vi "Patch data preview core.vi"(6 "Global cycle number among all trials":i32, 9 "Channel to load":enum16{"Red", "Green"}(ring)) -> (1 "Image ref (montage)":T1, 3 "Next state":T2=enum."Idle")   [LabVIEW 2017]
uses:
  Typedefs/Patch viewer internal cluster.ctl
  <vilib>/vision/Image Controls.llb/IMAQ Image.ctl
  Typedefs/Patch viewer states.ctl
  Typedefs/Read Write Enum.ctl
panel:
  out "Register cluster":T3
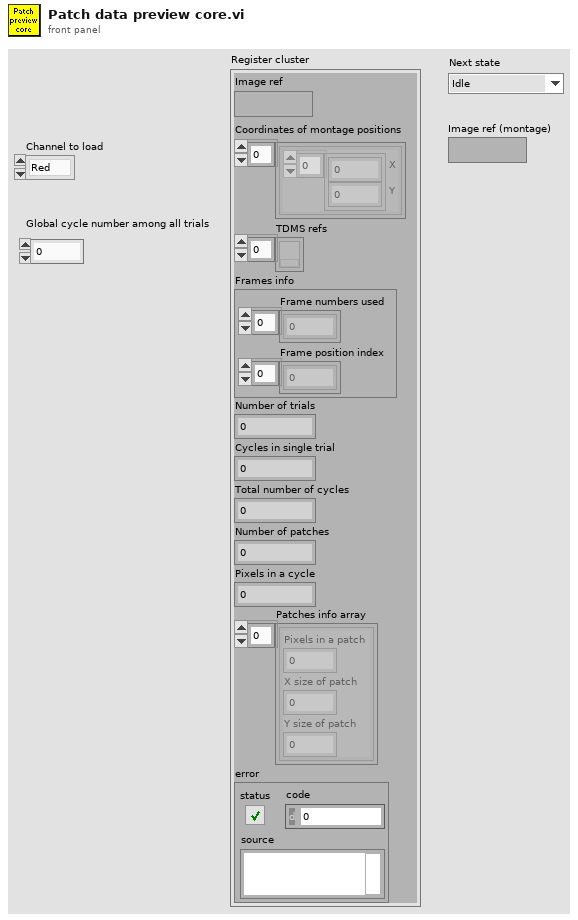
[diagram p1: front panel]
types:
  T1 = typedef "IMAQ Image.ctl" = refnum<image>
  T2 = typedef "Patch viewer states.ctl" = enum16{"Initialise", "Refresh", "Idle", "Error"}
  T3 = typedef "Patch viewer internal cluster.ctl" = cluster{"Image ref":T1, "Coordinates of montage positions":cluster{"X\n\nY":i32[]}[], "TDMS refs":refnum<k34>[], "Frames info":cluster{"Frame numbers used":i32[], "Frame position index":i32[]}, "Number of trials":i32, "Cycles in single trial":i32, "Total number of cycles":i32, "Number of patches":i32, "Pixels in a cycle":i32, "Patches info array":cluster{"Pixels in a patch":i32, "X size of patch":i32, "Y size of patch":i32}[], "error":errorcluster}
  T4 = typedef "Read Write Enum.ctl" = enum16{"Read", "Write"}
  T5 = typedef "Image Type" = u32
  T6 = cluster{"Frame numbers used":i32[], "Frame position index":i32[]}
  T7 = cluster{"Pixels in a patch":i32, "X size of patch":i32, "Y size of patch":i32}[]
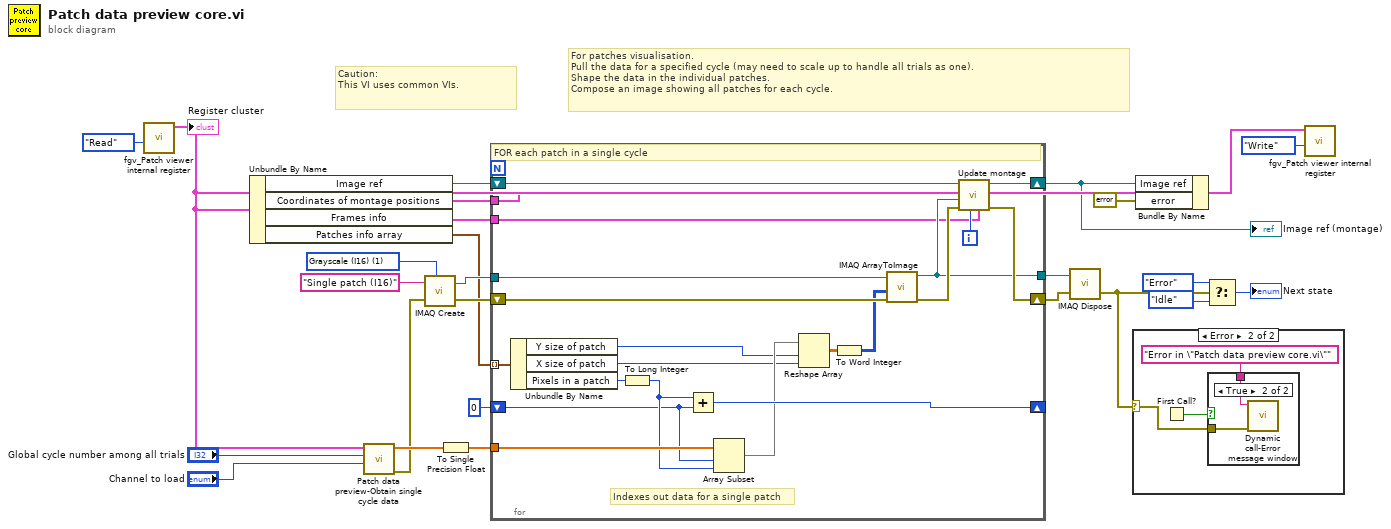
[diagram p0: block diagram]
diagram:
  w25 = T5 1 items=["Grayscale (U8)", "Grayscale (I16)", "Grayscale (SGL)", "Complex (CSG)", "RGB (U32)", "HSL (U32)", "RGB (U64)", "Grayscale (U16)"] ("Image Type")
  # "Caution:\nThis VI uses common VIs."
  # "For patches visualisation.\nPull the data for a specified cycle (may need to scale up to handle all trials as one).\nShape the data in the individual patches.\nCompose an image showing all patches for each cycle."
  n1 = call "fgv_Patch viewer internal register.vi"("Function"=Read_Write_Enum."Read") -> ("Registered setup"=w6:T3)  [unwired: 10 in]
  "Register cluster" <- w6
  n2 = Unbundle By Name(w6) -> ("Image ref"=w16:T1, "Coordinates of montage positions"=w15:cluster{"X\n\nY":i32[]}[], "Frames info"=w14:T6, "Patches info array"=w13:T7)
  n3 = call "Patch data preview-Obtain single cycle data.vi"("Channel to load"="Channel to load", "Global cycle number among all trials"="Global cycle number among all trials", "Register cluster"=w6) -> ("error out"=w17:errorcluster, "Data from single channel single cycle"=w20:dbl[])  [unwired: 7 in]
  n4 = call "IMAQ Create"("Image Name"="Single patch (I16)", "Image Type"=w25, "error in (no error)"=w17) -> ("New Image"=w23:T1, "error out"=w21:errorcluster)  [unwired: 1 in, 1 out]
  n5 = To Single Precision Float(number=w20) -> (single precision float=w22:sgl[])
  n6 = for {
    tunnel: w13 -> [w47] mode=indexing
    shift-right: [w44] -> _
    shift-left: 0 -> [w29]
    tunnel: w22 -> [w45]
    tunnel: w23 -> [w39]
    tunnel: [w32] -> w19
    shift-right: [w34] -> w18
    shift-left: w21 -> [w38]
    shift-right: [w30] -> w1
    shift-left: w16 -> [w36]
    tunnel: w15 -> [w37]
    tunnel: w14 -> [w31]
    i -> [w33]
    # "Indexes out data for a single patch"
    # "FOR each patch in a single cycle"
    n7 = Unbundle By Name(w47) -> ("Y size of patch"=w41:i32, "X size of patch"=w40:i32, "Pixels in a patch"=w46:i32)
    n8 = To Long Integer(number=w46) -> (32bit integer=w43:i32)
    n9 = Add(x=w43, y=w29) -> (x+y=w44:i32)
    n10 = Array Subset "Array Subset"(array=w45, index=w29, length=w43) -> (w42:sgl[])
    n11 = Reshape Array(w42, w41, w40) -> (w27:sgl[][])
    n12 = To Word Integer(number=w27) -> (16bit integer=w28:i16[][])
    n13 = call "IMAQ ArrayToImage"("error in (no error)"=w38, "Image Pixels (I16)"=w28, "Image"=w39) -> ("error out"=w35:errorcluster, "Image Out"=w32:T1)  [unwired: 7 in]
    n14 = call "Update montage.vi"("Frames info"=w31, "Frame's rel. index"=w33, "Error in"=w35, "Single patch image"=w32, "Coordinates of montage positions"=w37, "Image (Montage)"=w36) -> ("error out"=w34:errorcluster, "Image (Montage)"=w30:T1)  [unwired: 4 in]
  }
  "Image ref (montage)" <- w1
  n15 = call "IMAQ Dispose"("Image"=w19, "error in (no error)"=w18) -> ("error out"=w2:errorcluster)  [unwired: 4 in]
  n16 = case shown="Error" w2 {
    selector: w2 -> [_ w49]
    frame No Error {
    }
    frame Error {
      n17 = First Call?() -> (First Call?: T/F=w50:bool)
      n18 = case shown="True" w50 {
        tunnel: w49 -> [_ w52]
        tunnel: "Error in \"Patch data preview core.vi\"" ("Error Message") -> [_ w51]
        frame False {
        }
        frame True {
          n19 = call "Dynamic call-Error message window.vi"("error in (no error)"=w52, "Error Message"=w51) -> ()  [unwired: 9 in, 1 out]
        }
      }
    }
  }
  n20 = Bundle By Name(cluster=w6, "Image ref"=w1, "error"=errorcluster {"status"=FALSE, "code"=0, "source"=""}) -> (w4:T3)
  n21 = Select(t=Patch_viewer_states."Error" ("States"), s=w2, f=Patch_viewer_states."Idle" ("States")) -> (s? t:f=→"Next state":T2)
  n22 = call "fgv_Patch viewer internal register.vi"("Function"=Read_Write_Enum."Write", "Registered setup"=w4) -> ()  [unwired: 9 in, 1 out]
